vi "Create TreeNodeBox.vi"(1 "Pmin":sgl[](array[numeric]), 2 "Pmax":sgl[](array[numeric]), 3 "Parent":i32=-1, 4 "Level":i32=-1) -> (0 "Box":T1={"Face 0"={"V0"=[], "V1"=[], "V2"=[], "V3"=[], "E0"=[], "E1"=[], "E2"=[], "E3"=[], "n^"=[], "nE0^"=[], "nE1^"=[], "nE2^"=[], "nE3^"=[]}, "Face 1"={"V0"=[], "V1"=[], "V2"=[], "V3"=[], "E0"=[], "E1"=[], "E2"=[], "E3"=[], "n^"=[], "nE0^"=[], "nE1^"=[], "nE2^"=[], "nE3^"=[]}, "Face 2"={"V0"=[], "V1"=[], "V2"=[], "V3"=[], "E0"=[], "E1"=[], "E2"=[], "E3"=[], "n^"=[], "nE0^"=[], "nE1^"=[], "nE2^"=[], "nE3^"=[]}, "Face 3"={"V0"=[], "V1"=[], "V2"=[], "V3"=[], "E0"=[], "E1"=[], "E2"=[], "E3"=[], "n^"=[], "nE0^"=[], "nE1^"=[], "nE2^"=[], "nE3^"=[]}, "Face 4"={"V0"=[], "V1"=[], "V2"=[], "V3"=[], "E0"=[], "E1"=[], "E2"=[], "E3"=[], "n^"=[], "nE0^"=[], "nE1^"=[], "nE2^"=[], "nE3^"=[]}, "Face 5"={"V0"=[], "V1"=[], "V2"=[], "V3"=[], "E0"=[], "E1"=[], "E2"=[], "E3"=[], "n^"=[], "nE0^"=[], "nE1^"=[], "nE2^"=[], "nE3^"=[]}, "Level"=-1, "Pmax"=[], "Pmin"=[], "Parent"=-1, "Child 1"=-1, "Child 2"=-1, "Child 3"=-1, "Child 4"=-1, "Child 5"=-1, "Child 6"=-1, "Child 7"=-1, "Child 8"=-1, "Triangles"=[], "is leaf node"=FALSE})   [LabVIEW 2014]
uses:
  Typedefs/TreeNodeBox.ctl
  Typedefs/Quad.ctl
panel:
  # "PN 17/01/2015"
  # "Vertices"
  # "Edges"
  # "Unit normal"
  # "Edge unit normals"
  # "Vertices"
  # "Edges"
  # "Unit normal"
  # "Edge unit normals"
  # "Vertices"
  # "Edges"
  # "Unit normal"
  # "Edge unit normals"
  # "Vertices"
  # "Edges"
  # "Unit normal"
  # "Edge unit normals"
  # "Vertices"
  # "Edges"
  # "Unit normal"
  # "Edge unit normals"
  # "Vertices"
  # "Edges"
  # "Unit normal"
  # "Edge unit normals"
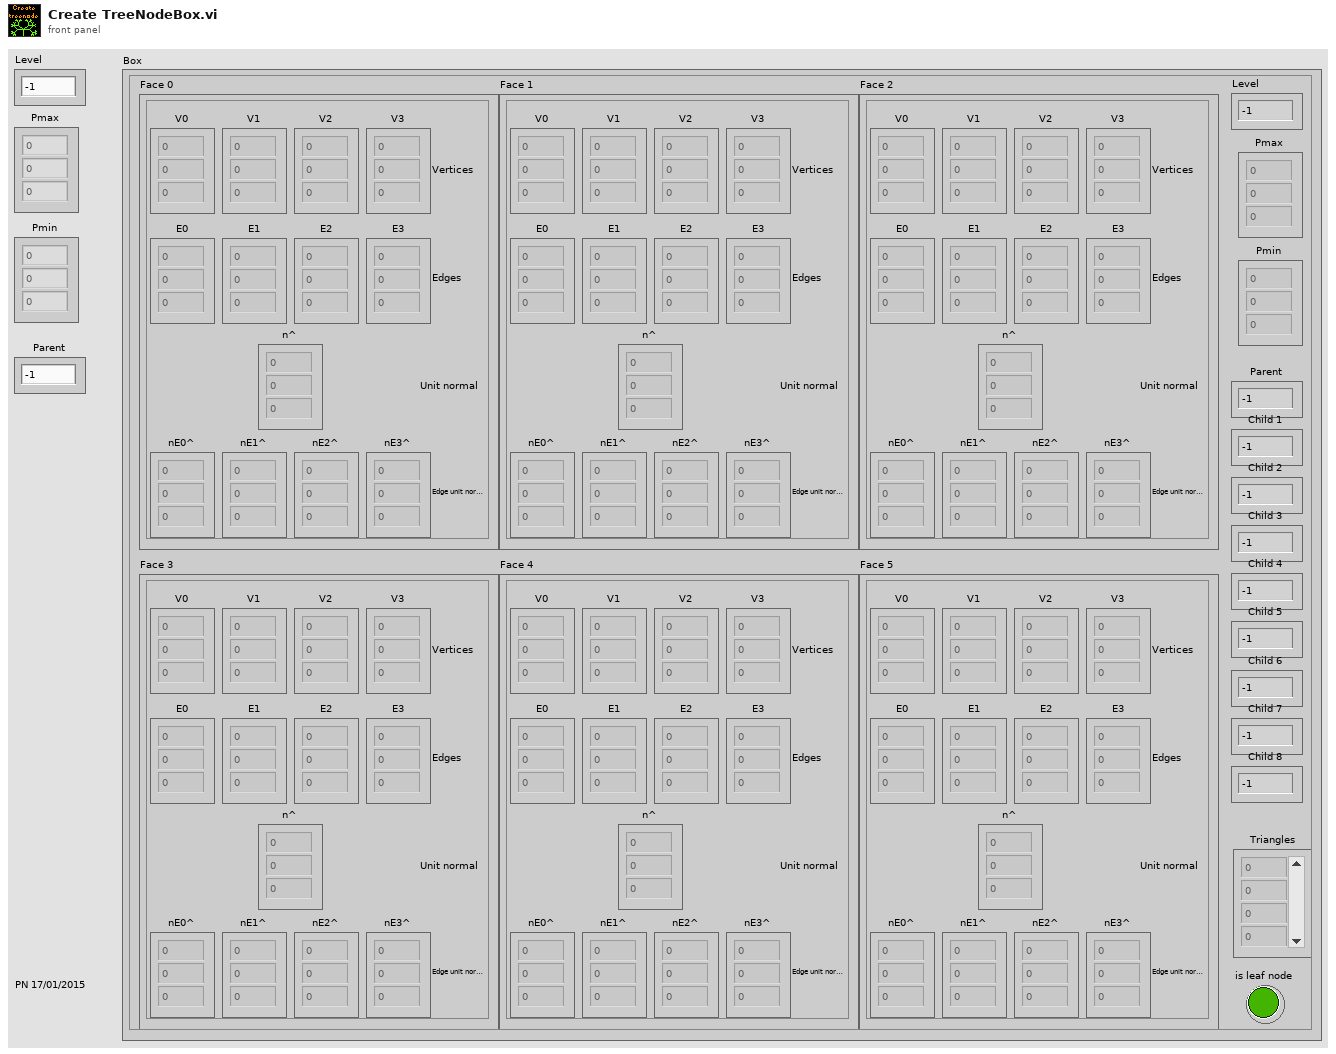
[diagram p1: front panel]
types:
  T1 = typedef "TreeNodeBox.ctl" = cluster{"Face 0":T2, "Face 1":T2, "Face 2":T2, "Face 3":T2, "Face 4":T2, "Face 5":T2, "Level":i32, "Pmax":sgl[], "Pmin":sgl[], "Parent":i32, "Child 1":i32, "Child 2":i32, "Child 3":i32, "Child 4":i32, "Child 5":i32, "Child 6":i32, "Child 7":i32, "Child 8":i32, "Triangles":i32[], "is leaf node":bool}
  T2 = typedef "Quad.ctl" = cluster{"V0":sgl[], "V1":sgl[], "V2":sgl[], "V3":sgl[], "E0":sgl[], "E1":sgl[], "E2":sgl[], "E3":sgl[], "n^":sgl[], "nE0^":sgl[], "nE1^":sgl[], "nE2^":sgl[], "nE3^":sgl[]}
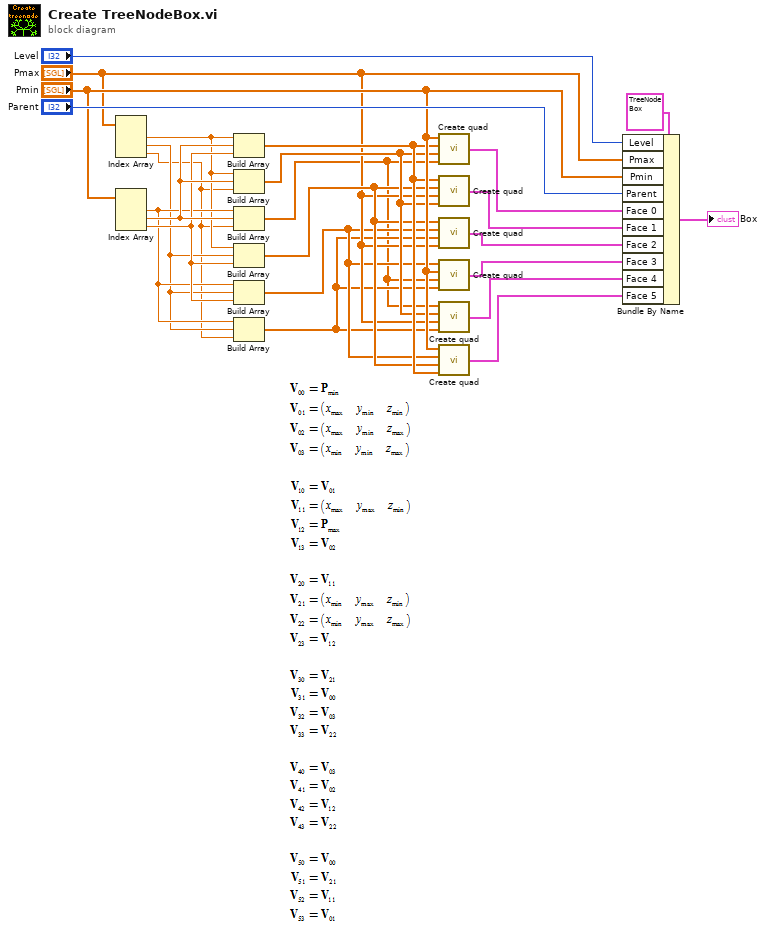
[diagram p0: block diagram]
diagram:
  n1 = Index Array(array="Pmax") -> (element #1=w5:sgl, element #2=w6:sgl, element #3=w1:sgl)  [unwired: 3 in]
  n2 = Index Array(array="Pmin") -> (element #1=w7:sgl, element #2=w12:sgl, element #3=w9:sgl)  [unwired: 3 in]
  n3 = Build Array(w5, w12, w9) -> (w14:sgl[])
  n4 = Build Array(w5, w12, w1) -> (w13:sgl[])
  n5 = Build Array(w7, w12, w1) -> (w3:sgl[])
  n6 = Build Array(w5, w6, w9) -> (w11:sgl[])
  n7 = Build Array(w7, w6, w9) -> (w8:sgl[])
  n8 = Build Array(w7, w6, w1) -> (w4:sgl[])
  n9 = call "Create quad.vi"("V3"=w3, "V2"=w13, "V1"=w14, "V0"="Pmin") -> ("Quad"=w24:T2)
  n10 = call "Create quad.vi"("V3"=w13, "V2"="Pmax", "V1"=w11, "V0"=w14) -> ("Quad"=w23:T2)
  n11 = call "Create quad.vi"("V3"="Pmax", "V2"=w4, "V1"=w8, "V0"=w11) -> ("Quad"=w22:T2)
  n12 = call "Create quad.vi"("V3"=w4, "V2"=w3, "V1"="Pmin", "V0"=w8) -> ("Quad"=w21:T2)
  n13 = call "Create quad.vi"("V3"=w4, "V2"="Pmax", "V1"=w13, "V0"=w3) -> ("Quad"=w20:T2)
  n14 = call "Create quad.vi"("V3"=w14, "V2"=w11, "V1"=w8, "V0"="Pmin") -> ("Quad"=w19:T2)
  n15 = Bundle By Name(cluster=T1 {"Face 0"={"V0"=[], "V1"=[], "V2"=[], "V3"=[], "E0"=[], "E1"=[], "E2"=[], "E3"=[], "n^"=[], "nE0^"=[], "nE1^"=[], "nE2^"=[], "nE3^"=[]}, "Face 1"={"V0"=[], "V1"=[], "V2"=[], "V3"=[], "E0"=[], "E1"=[], "E2"=[], "E3"=[], "n^"=[], "nE0^"=[], "nE1^"=[], "nE2^"=[], "nE3^"=[]}, "Face 2"={"V0"=[], "V1"=[], "V2"=[], "V3"=[], "E0"=[], "E1"=[], "E2"=[], "E3"=[], "n^"=[], "nE0^"=[], "nE1^"=[], "nE2^"=[], "nE3^"=[]}, "Face 3"={"V0"=[], "V1"=[], "V2"=[], "V3"=[], "E0"=[], "E1"=[], "E2"=[], "E3"=[], "n^"=[], "nE0^"=[], "nE1^"=[], "nE2^"=[], "nE3^"=[]}, "Face 4"={"V0"=[], "V1"=[], "V2"=[], "V3"=[], "E0"=[], "E1"=[], "E2"=[], "E3"=[], "n^"=[], "nE0^"=[], "nE1^"=[], "nE2^"=[], "nE3^"=[]}, "Face 5"={"V0"=[], "V1"=[], "V2"=[], "V3"=[], "E0"=[], "E1"=[], "E2"=[], "E3"=[], "n^"=[], "nE0^"=[], "nE1^"=[], "nE2^"=[], "nE3^"=[]}, "Level"=-1, "Pmax"=[], "Pmin"=[], "Parent"=-1, "Child 1"=-1, "Child 2"=-1, "Child 3"=-1, "Child 4"=-1, "Child 5"=-1, "Child 6"=-1, "Child 7"=-1, "Child 8"=-1, "Triangles"=[], "is leaf node"=FALSE} ("Box"), "Level"="Level", "Pmax"="Pmax", "Pmin"="Pmin", "Parent"="Parent", "Face 0"=w24, "Face 1"=w23, "Face 2"=w22, "Face 3"=w21, "Face 4"=w20, "Face 5"=w19) -> (→"Box":T1)
